vi "Create Processing Payload.vi"(8 "error in (no error)":errorcluster, 11 "Settings in":T11 {"Processing Settings"."Test Parameters"."Allowed Tolerance (%) FS" format="%#_4g"; "Acq Settings"."Config Settings"."Simulated Sensor Injection" scale=0.0..100.0}) -> (0 "error out":errorcluster, 2 "Processing Settings":T1 {"Test Parameters"."Allowed Tolerance (%) FS" format="%#_4g"}, 3 "Settings out":T11 {"Processing Settings"."Test Parameters"."Allowed Tolerance (%) FS" format="%#_4g"; "Acq Settings"."Config Settings"."Simulated Sensor Injection" scale=0.0..100.0})   [LabVIEW 2026, in "Processing_Engine.lvlib"]
uses:
  Processing/Processing_Engine.lvlib
  controls/UI/Settings Cluster.ctl
  controls/UI/Acq Settings.ctl
  Acquisition/Instrument Specifications Configuration.ctl
  Acquisition/Instrument Specifications Cluster Configuration.ctl
  controls/UI/Measurement Role.ctl
  controls/UI/Config Settings.ctl
  Processing/Processing Settings.ctl
  controls/Messaging Payloads/Sensor CoreData.ctl
  controls/Messaging Payloads/Sensor CoreData Cluster.ctl
  controls/UI/Units Enum.ctl
  controls/UI/Signal Enum.ctl
  Processing/Test Parameters.ctl
  Processing/Test Parameters Cluster.ctl
  controls/UI/Test Sequence Context.ctl
  controls/UI/Direction.ctl
  controls/UI/Session Identfiers.ctl
  controls/UI/Test Sequence Settings.ctl
  controls/UI/Test Sequence State.ctl
  controls/UI/Test Sequence Enum.ctl
  controls/Controller/Stimulus Settings.ctl
  controls/Controller/Stimulus Outputs.ctl
  controls/Controller/Stimulus Output.ctl
  controls/Controller/Controller Core Data.ctl
  controls/Controller/Stimulus Output Configuration.ctl
  controls/Controller/Stimulus Role.ctl
  controls/UI/Test Sequence Context Cluster.ctl
  Settings/Settings.lvlib
  Acquisition/Acquisition.lvlib
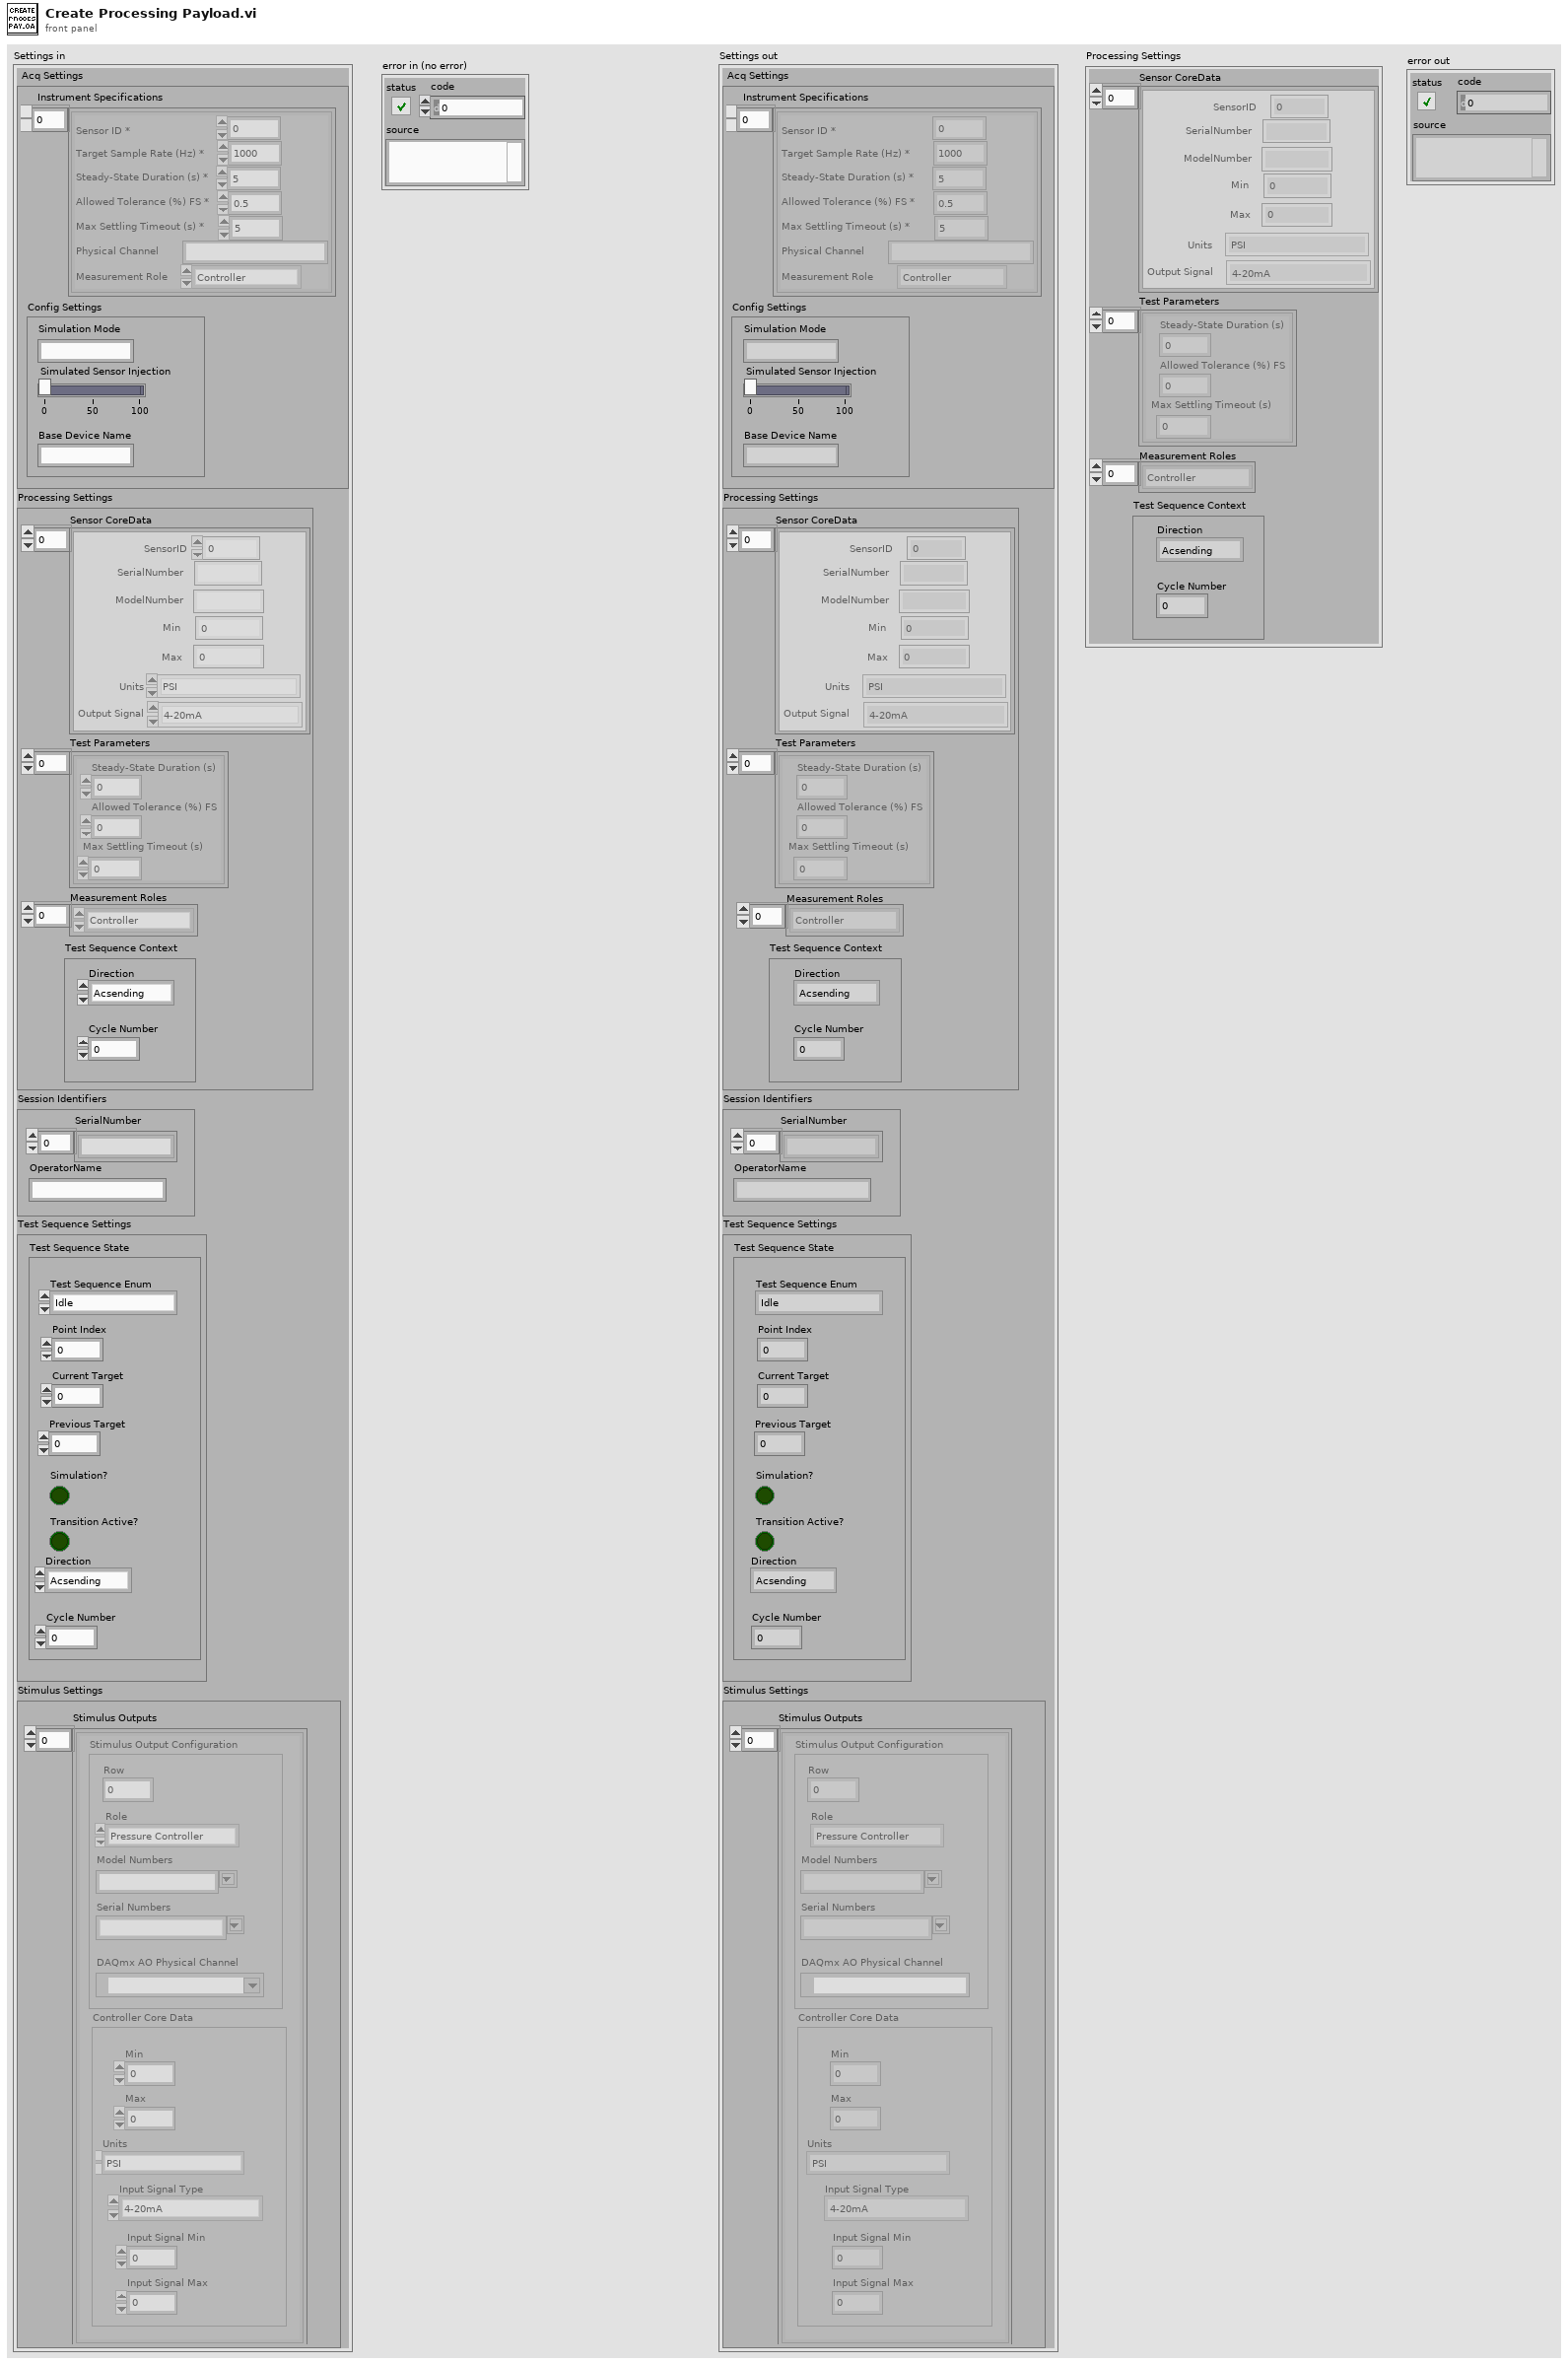
[diagram p1: front panel]
types:
  T1 = typedef "Processing_Engine.lvlib/Processing Settings.ctl" = cluster{"Sensor CoreData":T2, "Test Parameters":T6, "Measurement Roles":T8[], "Test Sequence Context":T9}
  T2 = typedef "Sensor CoreData.ctl" = T3[]
  T3 = typedef "Settings.lvlib/Sensor CoreData Cluster.ctl" = cluster{"SerialNumber":string, "ModelNumber":string, "Min":dbl, "Max":dbl, "Units":T4, "Output Signal":T5, "SensorID":i32}
  T4 = typedef "Units Enum.ctl" = enum16{"PSI", "Deg C", "kPa", "GPM"}
  T5 = typedef "Signal Enum.ctl" = enum16{"4-20mA", "0-10V", "Thermocouple Type K"}
  T6 = typedef "Processing_Engine.lvlib/Test Parameters.ctl" = T7[]
  T7 = typedef "Settings.lvlib/Test Parameters Cluster.ctl" = cluster{"Steady-State Duration (s)":i32, "Allowed Tolerance (%) FS":dbl, "Max Settling Timeout (s)":i32}
  T8 = typedef "Settings.lvlib/Measurement Role.ctl" = enum16{"Controller", "Reference", "UUT", "Disable", "All"}
  T9 = typedef "Settings.lvlib/Test Sequence Context.ctl" = cluster{"Direction":T10, "Cycle Number":i32}
  T10 = typedef "Settings.lvlib/Direction.ctl" = enum16{"Acsending", "Descending"}
  T11 = typedef "Settings Cluster.ctl" = cluster{"Acq Settings":T12, "Processing Settings":T1, "Session Identifiers":T16, "Test Sequence Settings":T17, "Stimulus Settings":T20}
  T12 = typedef "Acq Settings.ctl" = cluster{"Instrument Specifications":T13, "Config Settings":T15}
  T13 = typedef "Acquisition.lvlib/Instrument Specifications Configuration.ctl" = T14[]
  T14 = typedef "Acquisition.lvlib/Instrument Specifications Cluster Configuration.ctl" = cluster{"Sensor ID *":i32, "Target Sample Rate (Hz) *":dbl, "Steady-State Duration (s) *":i32, "Allowed Tolerance (%) FS *":dbl, "Max Settling Timeout (s) *":i32, "Physical Channel":string, "Measurement Role":T8}
  T15 = typedef "Config Settings.ctl" = cluster{"Simulated Sensor Injection":dbl, "Base Device Name":string, "Simulation Mode":string}
  T16 = typedef "Session Identfiers.ctl" = cluster{"SerialNumber":string[], "OperatorName":string}
  T17 = typedef "Test Sequence Settings.ctl" = cluster{"Test Sequence State":T18}
  T18 = typedef "Settings.lvlib/Test Sequence State.ctl" = cluster{"Test Sequence Enum":T19, "Point Index":i32, "Current Target":dbl, "Previous Target":dbl, "Simulation?":bool, "Direction":T10, "Transition Active?":bool, "Cycle Number":i32}
  T19 = typedef "Test Sequence Enum.ctl" = enum16{"Idle", "Start Point", "Point Complete", "Test Complete", "Abort Test", "Reset"}
  T20 = typedef "Settings.lvlib/Stimulus Settings.ctl" = cluster{"Stimulus Outputs":T21}
  T21 = typedef "Settings.lvlib/Stimulus Outputs.ctl" = T22[]
  T22 = typedef "Settings.lvlib/Stimulus Output.ctl" = cluster{"Controller Core Data":T23, "Stimulus Output Configuration":T24}
  T23 = typedef "Settings.lvlib/Controller Core Data.ctl" = cluster{"Min":dbl, "Max":dbl, "Units":T4, "Input Signal Type":T5, "Input Signal Min":dbl, "Input Signal Max":dbl}
  T24 = typedef "Settings.lvlib/Stimulus Output Configuration.ctl" = cluster{"DAQmx AO Physical Channel":tag, "Role":T25, "Model Numbers":string, "Serial Numbers":string, "Row":i32}
  T25 = typedef "Stimulus Role.ctl" = enum16{"Pressure Controller", "Temperature Controller"}
  T26 = typedef "Settings.lvlib/Test Sequence Context Cluster.ctl" = cluster{"Direction":T10, "Cycle Number":i32}
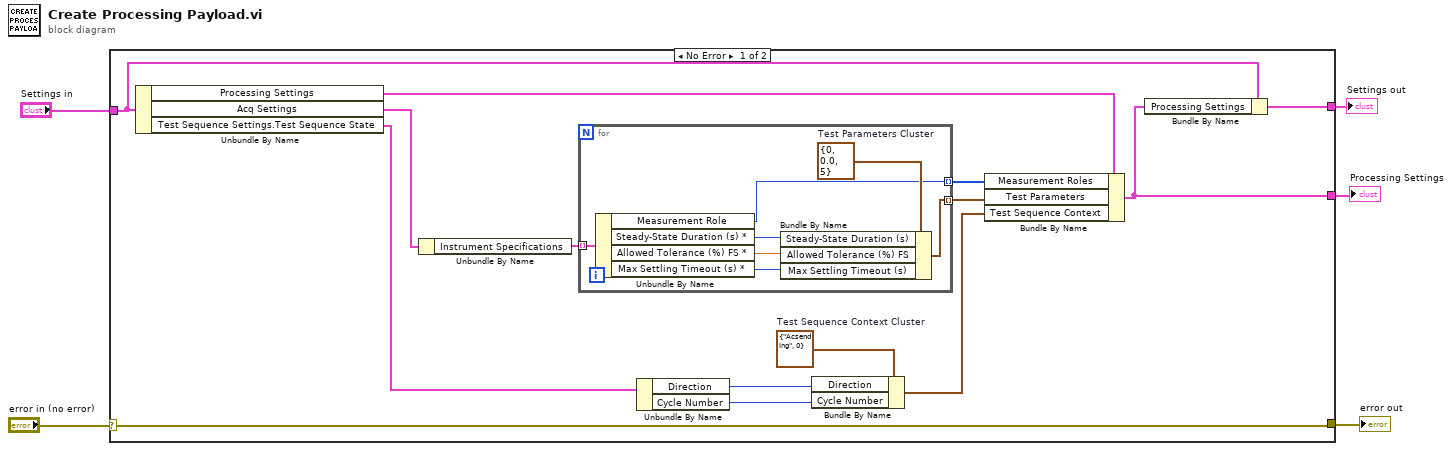
[diagram p0: block diagram]
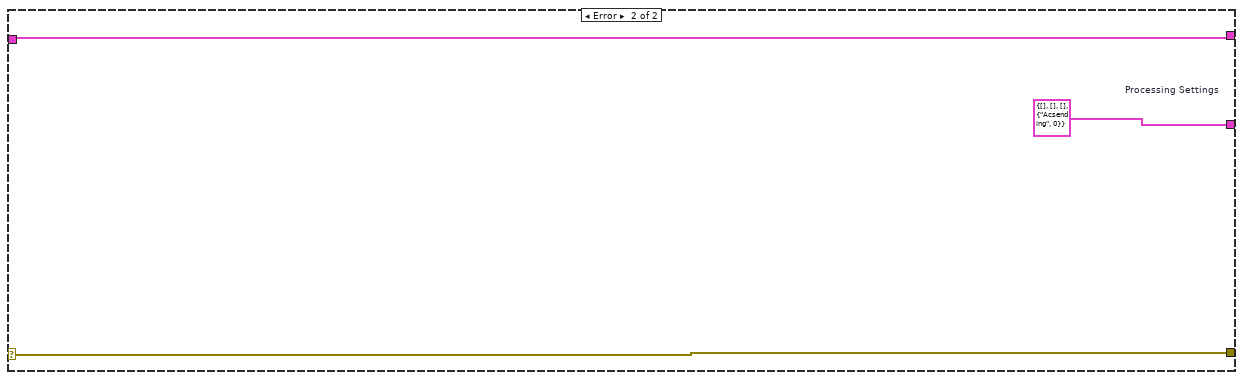
[diagram p2: hidden frame]
diagram:
  n1 = case shown="No Error" "error in (no error)" {
    selector: "error in (no error)" -> [w13 w28]
    tunnel: [w19 w29] -> w5
    tunnel: "Settings in" -> [w11 w29]
    tunnel: [w13 w28] -> w2
    tunnel: [w12 w27] -> w1
    frame No Error {
      w10 = T26 {"Direction"=enum."Acsending", "Cycle Number"=0}  # Test Sequence Context Cluster
      n2 = Unbundle By Name(w11) -> ("Processing Settings"=w15:T1, "Acq Settings"=w16:T12, "Test Sequence Settings.Test Sequence State"=w7:T18)
      n3 = Unbundle By Name(w16) -> ("Instrument Specifications"=w18:T13)
      n4 = for {
        tunnel: [w26] -> w17 mode=indexing
        tunnel: w18 -> [w25] mode=indexing
        tunnel: [w20] -> w14 mode=indexing
        w21 = T7 {"Steady-State Duration (s)"=0, "Allowed Tolerance (%) FS"=0.0, "Max Settling Timeout (s)"=5}  # Test Parameters Cluster
        n5 = Unbundle By Name(w25) -> ("Measurement Role"=w20:T8, "Steady-State Duration (s) *"=w24:i32, "Allowed Tolerance (%) FS *"=w23:dbl, "Max Settling Timeout (s) *"=w22:i32)
        n6 = Bundle By Name(cluster=w21, "Steady-State Duration (s)"=w24, "Allowed Tolerance (%) FS"=w23, "Max Settling Timeout (s)"=w22) -> (w26:T7)
      }
      n7 = Unbundle By Name(w7) -> ("Direction"=w9:T10, "Cycle Number"=w8:i32)
      n8 = Bundle By Name(cluster=w10, "Direction"=w9, "Cycle Number"=w8) -> (w6:T26)
      n9 = Bundle By Name(cluster=w15, "Measurement Roles"=w14, "Test Parameters"=w17, "Test Sequence Context"=w6) -> (w12:T1)
      n10 = Bundle By Name(cluster=w11, "Processing Settings"=w12) -> (w19:T11)
    }
    frame Error {
      w27 = T1 {"Sensor CoreData"=[], "Test Parameters"=[], "Measurement Roles"=[], "Test Sequence Context"={"Direction"=enum."Acsending", "Cycle Number"=0}}  # Processing Settings
    }
  }
  "Settings out" <- w5
  "error out" <- w2
  "Processing Settings" <- w1
